vi "MPX Fill Sequence Selectors.vi"(8 "error in":errorcluster, 10 "Strings []":string[](array[string]), 11 "transducer list ref":refnum<vi>) -> (0 "error out":errorcluster, 3 "transducer list ref out":refnum<vi>)   [LabVIEW 2013]
doc: "Fills the channel selector in the array of sequence items by given strings."
uses:
  measure/Corrections/Corr Tranducer ADC Channel.ctl
panel:
  in  "Ring":T1
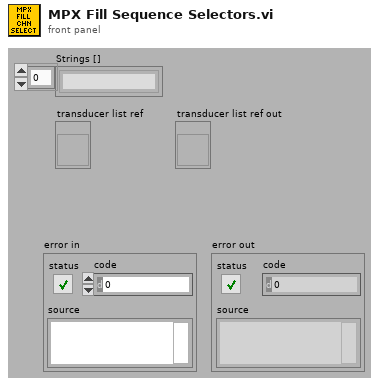
[diagram p1: front panel]
types:
  T1 = typedef "Corr Tranducer ADC Channel.ctl" = u16
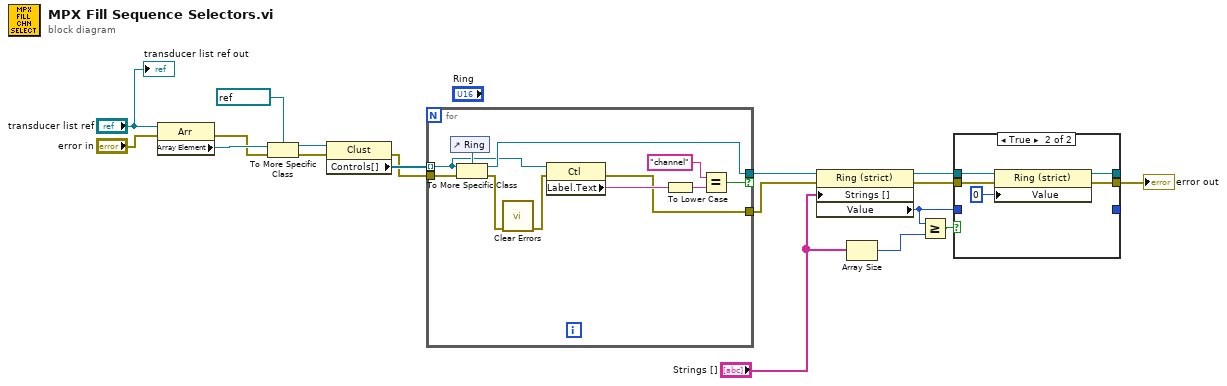
[diagram p0: block diagram]
diagram:
  n1 = property class="Arr"(reference="transducer list ref", error in="error in") -> (error out=w17:errorcluster, "Array Element"=w18:refnum<vi>)  [unwired: 1 out]
  n2 = To More Specific Class(target class=refnum<vi> refnum ("Cluster"), reference=w18, error in=w17) -> (specific class reference=w15:refnum<vi>, error out=w16:errorcluster)
  n3 = property class="Clust"(reference=w15, error in=w16) -> (error out=w12:errorcluster, "Controls[]"=w14:refnum<vi>[])  [unwired: 1 out]
  n4 = for {
    tunnel: w14 -> [w21] mode=indexing
    tunnel: [w23] -> w5 if=w25
    tunnel: [w27] -> w6
    tunnel: w12 -> [w24]
    n5 = control-ref of="Ring"() -> (w22:refnum<vi>)
    n6 = To More Specific Class(target class=w22, reference=w21, error in=w24) -> (specific class reference=w23:refnum<vi>, error out=w20:errorcluster)
    n7 = call <vilib>:"Clear Errors.vi"("error in (no error)"=w20) -> ("error out"=w19:errorcluster)  [unwired: 6 in]
    n8 = property class="Ctl"(reference=w21, error in=w19) -> (error out=w27:errorcluster, "Label.Text"=w28:string)  [unwired: 1 out]
    n9 = To Lower Case(string=w28) -> (all lower case string=w26:string)
    n10 = Equal?(x="channel", y=w26) -> (x = y?=w25:bool)
  }
  n11 = property class="Ring (strict)"(reference=w5, error in=w6, "Strings []"="Strings []") -> (reference out=w9:refnum<vi>, error out=w10:errorcluster, "Value"=w7:T1)
  n12 = Array Size(array="Strings []") -> (size(s)=w11:i32)
  n13 = Greater Or Equal?(x=w7, y=w11) -> (x >= y?=w8:bool)
  n14 = case shown="True" w8 {
    tunnel: w10 -> [w32 w37]
    tunnel: w9 -> [w31 w36]
    tunnel: [w32 w34] -> w1
    tunnel: [w31 w33] -> _
    tunnel: w7 -> [w30 _]
    tunnel: [w30 _] -> _
    frame False {
    }
    frame True {
      n15 = property class="Ring (strict)"(reference=w36, error in=w37, "Value"=u16 0) -> (reference out=w33:refnum<vi>, error out=w34:errorcluster)
    }
  }
  "error out" <- w1
  "transducer list ref out" <- "transducer list ref"
